vi "Time Remaining Control.vi"(10 "Numeric":dbl, 11 "Mode":enum16{"Get", "Set"}(ring)) -> (2 "Time Remaining":dbl)   [LabVIEW 2013]
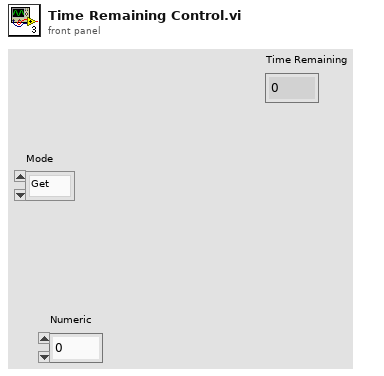
[diagram p1: front panel]
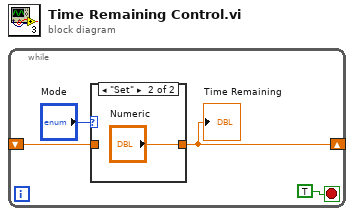
[diagram p0: block diagram]
diagram:
  n1 = while {
    shift-right: [w2] -> _
    shift-left: _ -> [w1]
    stop <- TRUE stop-if-true
    n2 = case shown="\"Set\"" "Mode" {
      tunnel: [w5 "Numeric"] -> w2
      tunnel: w1 -> [w5 _]
      frame "Get", Default {
      }
      frame "Set" {
      }
    }
    "Time Remaining" <- w2
  }
